vi "Final_LP2.vi"() -> ()   [LabVIEW 2017]
panel:
  out "Waveform Chart":cluster{"TEM1":dbl, "TEM2":dbl, "TEM2":dbl}(graph)
  out "IsOpen 3":bool
  out "Multicolumn Listbox":i32(listbox)
  out "LED 3":bool
  out "LED 2":bool
  out "LED 1":bool
  in  "PUERTO":string(combo)
  in  "BaudRate":i32=9600
  in  "Close":bool
  in  "Open":bool
  in  "Umbral min3":dbl
  in  "Umbral max3":dbl
  in  "Umbral min2":dbl
  in  "Umbral max2":dbl
  in  "Umbral min1":dbl
  in  "Umbral max1":dbl
  out "lm35_3":dbl(knob) scale=0.0..150.0
  out "lm35_2":dbl(knob) scale=0.0..150.0
  out "lm35":dbl(knob) scale=0.0..150.0
  out "Sensor3_Dec":dbl
  out "Sensor2_Dec":dbl
  out "Sensor1_Dec":dbl
  out "element":string
  out "Datos":string
  out "BytesToRead":i32
  in  "STOP":bool
  # "PRUEBAS"
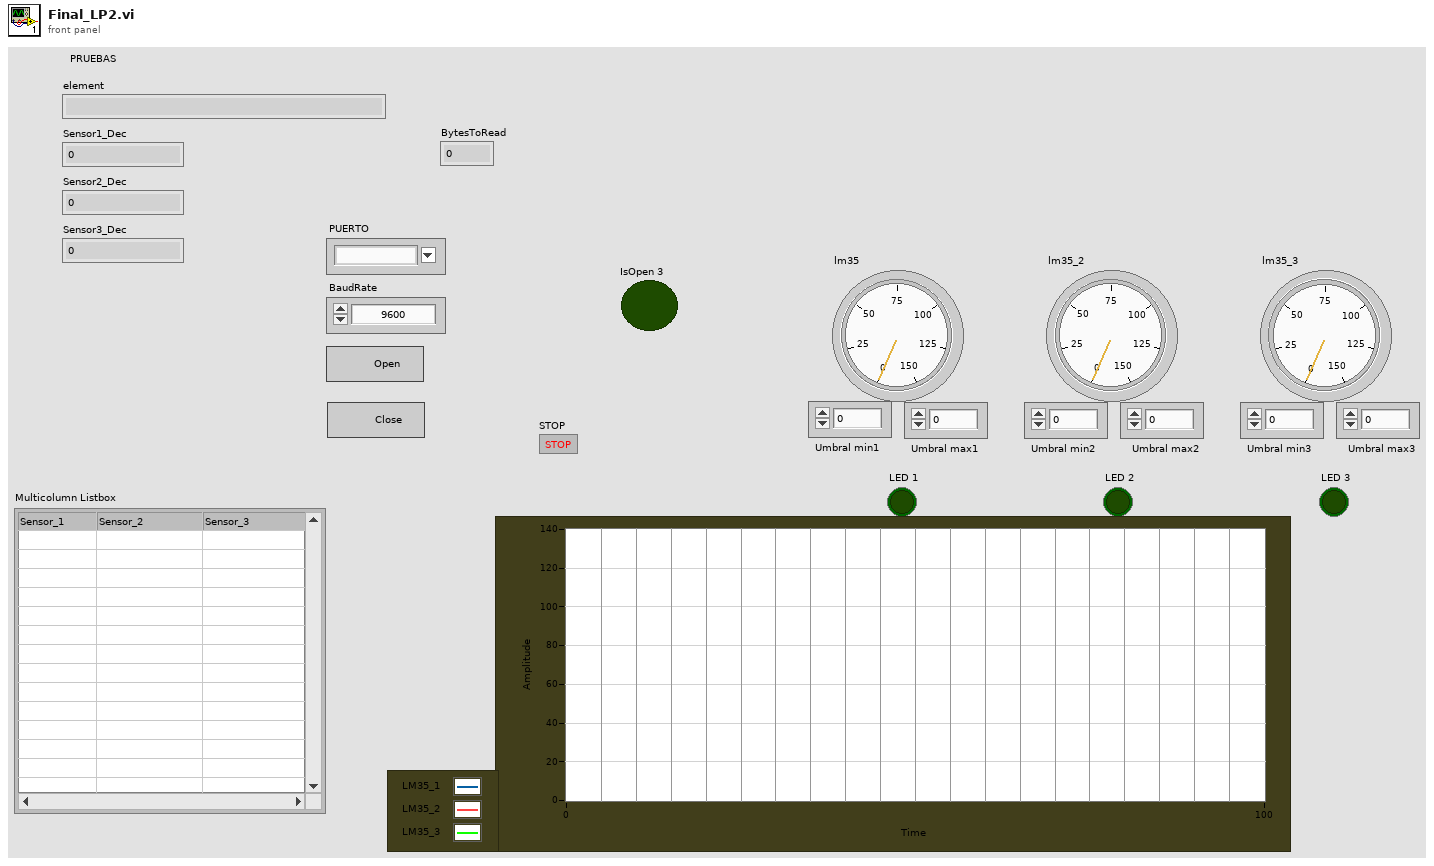
[diagram p1: front panel]
types:
  T1 = enum16{"open", "replace", "create", "open or create", "replace or create", "replace or create with confirmation"}
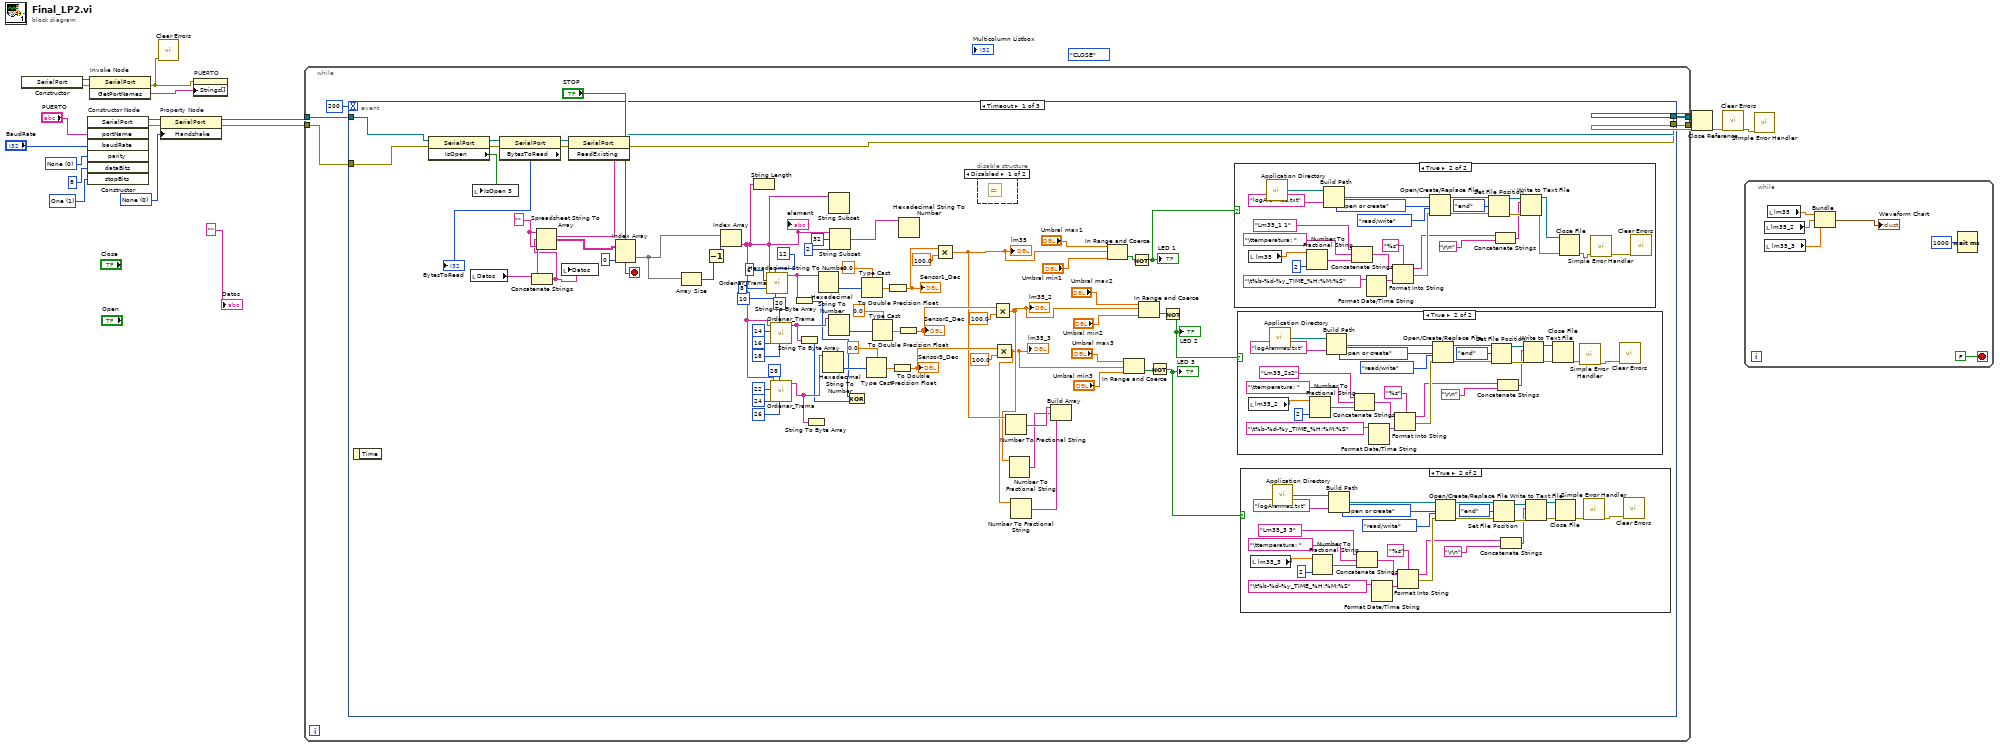
[diagram p0: block diagram]
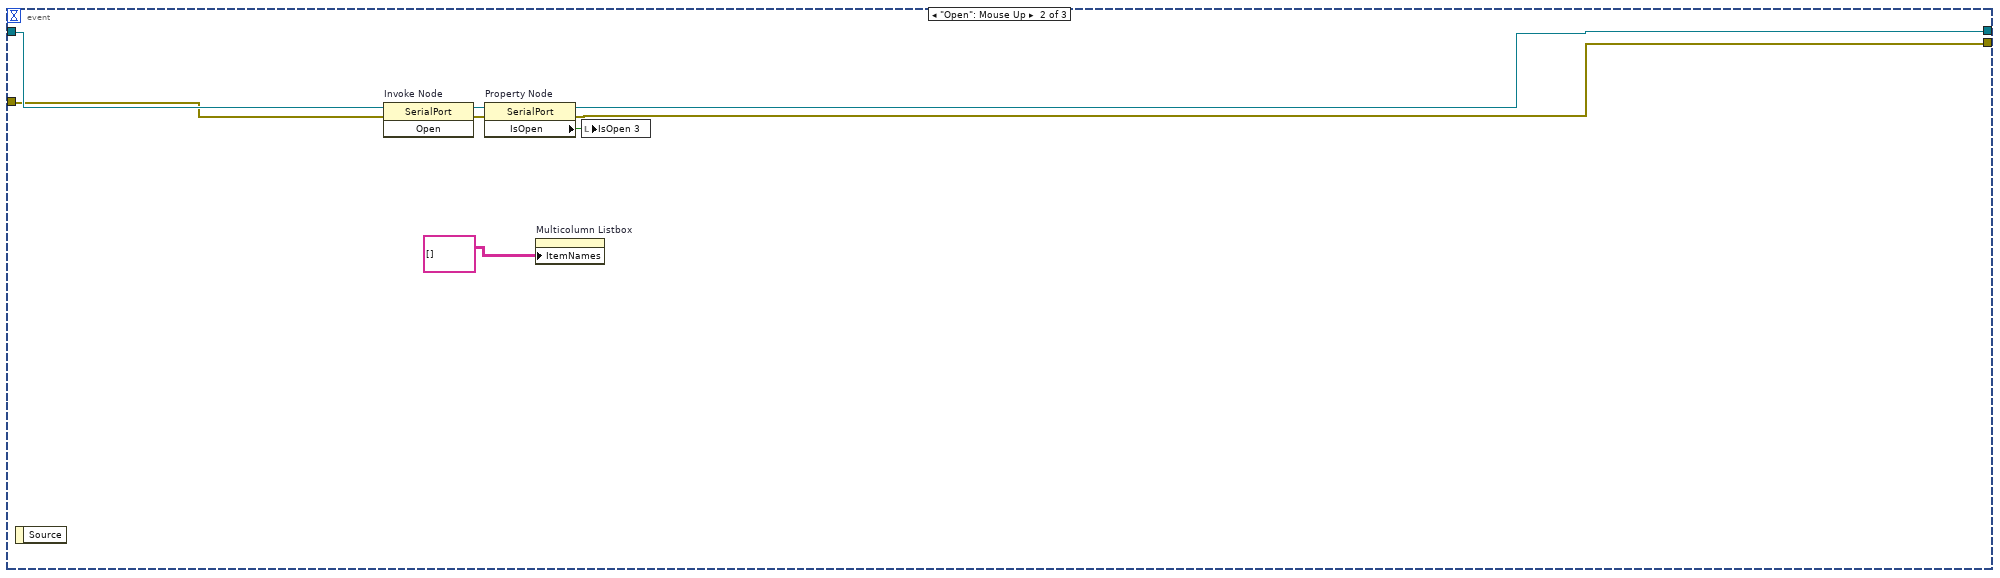
[diagram p6: hidden frame]
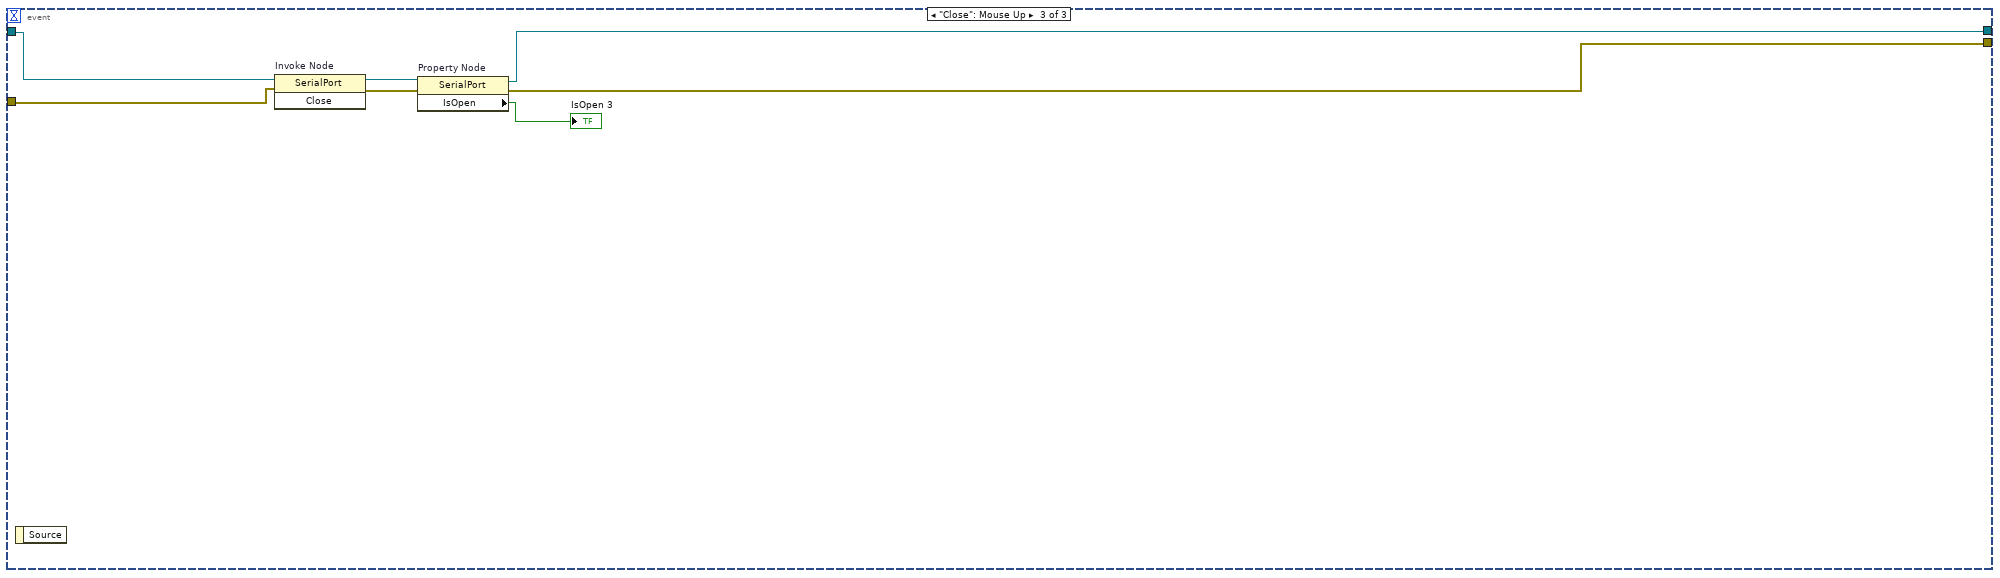
[diagram p7: hidden frame]
diagram:
  (unwired) enum16{"OPEN", "CLOSE", "READ"}."CLOSE"
  w10 = 1 items=["None", "One", "Two", "OnePointFive"] ("stopBits")
  w13 = 0 items=["None", "XOnXOff", "RequestToSend", "RequestToSendXOnXOff"] ("Handshake")
  w12 = 0 items=["None", "Odd", "Even", "Mark", "Space"] ("parity")
  n1 = constructor class="SerialPort"() -> (reference out=w17:refnum<k24>, error out=w16:errorcluster)  [unwired: 3 in, 1 out]
  n2 = constructor on="Constructor Node" class="SerialPort"("portName"="PUERTO", "baudRate"="BaudRate", "parity"=w12, "dataBits"=8, "stopBits"=w10) -> (reference out=w15:refnum<k24>, error out=w14:errorcluster)  [unwired: 3 in, 6 out]
  n3 = invoke on="Invoke Node" class="SerialPort" method="GetPortNames"(reference=w17, error in=w16) -> (error out=w7:errorcluster, "GetPortNames"=w8:string[])  [unwired: 1 in, 1 out]
  n4 = call <vilib>:"Clear Errors.vi"("error in (no error)"=w7) -> ()  [unwired: 5 in, 2 out]
  n5 = property on="Property Node" class="SerialPort"(reference=w15, error in=w14, "Handshake"=w13) -> (reference out=w5:refnum<k24>, error out=w4:errorcluster)
  n6 = property on="PUERTO" class="CmbBox"(error in=w7, "Strings[]"=w8) -> ()  [unwired: 1 in, 2 out]
  n7 = while {
    tunnel: w5 -> [w25]
    tunnel: [w21] -> w3
    tunnel: w4 -> [w24]
    tunnel: [w20] -> w2
    stop <- "STOP" stop-if-true
    n8 = event shown="[0] Timeout" {
      selector: _ -> [_ _ _]
      dyn-events: _ -> [_ _ _]
      timeout: 200 -> [_ _ _]
      tunnel: [w98 w182 w189] -> w21
      tunnel: w25 -> [w97 w184 w191]
      tunnel: w24 -> [w96 w183 w190]
      tunnel: [w95 w181 w188] -> w20
      event Timeout {
        w91 = "" ("format string")
        n9 = event-data() -> ()  [unwired: 1 in, 1 out]
        n10 = property class="SerialPort"(reference=w97, error in=w96) -> (reference out=w42:refnum<k24>, error out=w41:errorcluster, "IsOpen"=w40:bool)
        n11 = local read "Datos"() -> (w89:string)
        n12 = local write "IsOpen 3"(w40) -> ()
        n13 = property class="SerialPort"(reference=w42, error in=w41) -> (reference out=w92:refnum<k24>, error out=w94:errorcluster, "BytesToRead"=→"BytesToRead":i32)
        n14 = invoke class="SerialPort" method="ReadExisting"(reference=w92, error in=w94) -> (reference out=w98:refnum<k24>, error out=w95:errorcluster, "ReadExisting"=w90:string)  [unwired: 1 in]
        n15 = Concatenate Strings(w89, w90) -> (w88:string)
        n16 = Spreadsheet String To Array(format string=w91, spreadsheet string=w88, array type (2D Dbl)=w91) -> (array=w87:string[][])  [unwired: 1 in]
        n17 = local write "Datos"(w88) -> ()
        n18 = Index Array(array=w87, index (col)=0 ("disabled index (col)")) -> (element=w85:string[])  [unwired: 1 in]
        n19 = Array Size(array=w85) -> (size(s)=w84:i32)
        n20 = Decrement(x=w84) -> (x-1=w83:i32)
        n21 = Index Array(array=w85, index=w83) -> (element=w43:string)
        "element" <- w43
        n22 = String Length(string=w43) -> ()  [unwired: 1 out]
        n23 = call "Ordenar_Trama.vi"("offset (0) 3"=10 ("offset (0)"), "offset (0) 4"=12 ("offset (0)"), "offset (0) 2"=8 ("offset (0)"), "offset (0) 1"=6 ("offset (0)"), "format string"=w43) -> ("String"=w39:string)  [unwired: 6 in]
        n24 = call "Ordenar_Trama.vi"("offset (0) 3"=18, "offset (0) 4"=20, "offset (0) 2"=16, "offset (0) 1"=14, "format string"=w43) -> ("String"=w38:string)  [unwired: 6 in]
        n25 = call "Ordenar_Trama.vi"("offset (0) 3"=26, "offset (0) 4"=28, "offset (0) 2"=24, "offset (0) 1"=22, "format string"=w43) -> ("String"=w37:string)  [unwired: 6 in]
        n26 = String To Byte Array(string=w39) -> (unsigned byte array=w36:u8[])
        n27 = String To Byte Array(string=w38) -> (unsigned byte array=w35:u8[])
        n28 = String To Byte Array(string=w37) -> ()  [unwired: 1 out]
        n29 = Hexadecimal String To Number(string=w39) -> (number=w70:u32)  [unwired: 2 in, 1 out]
        n30 = Hexadecimal String To Number(string=w37) -> (number=w64:u32)  [unwired: 2 in, 1 out]
        n31 = String Subset(string=w43) -> ()  [unwired: 2 in, 1 out]
        n32 = Hexadecimal String To Number(string=w38) -> (number=w65:u32)  [unwired: 2 in, 1 out]
        n33 = String Subset(string=w43, offset (0)=32, length (rest)=2 ("length (rest)")) -> (substring=w44:string)
        n34 = Exclusive Or(1:w35, 2:w36) -> ()  [unwired: 1 out]
        n35 = Type Cast(type=sgl 0.0, x=w70) -> (*(type *) &x=w68:sgl)
        n36 = Type Cast(type=sgl 0.0, x=w64) -> (*(type *) &x=w62:sgl)
        n37 = Type Cast(type=sgl 0.0, x=w65) -> (*(type *) &x=w67:sgl)
        n38 = To Double Precision Float(number=w68) -> (double precision float=w61:dbl)
        "Sensor1_Dec" <- w61
        n39 = To Double Precision Float(number=w62) -> (double precision float=w57:dbl)
        "Sensor3_Dec" <- w57
        n40 = To Double Precision Float(number=w67) -> (double precision float=w56:dbl)
        "Sensor2_Dec" <- w56
        n41 = Hexadecimal String To Number(string=w44) -> ()  [unwired: 2 in, 2 out]
        n42 = Multiply(x=w61, y=100.0) -> (x*y=w31:dbl)
        "lm35" <- w31
        n43 = disable-structure shown="Disabled" {
          frame Disabled {
            n44 = Equal?() -> ()  [unwired: 2 in, 1 out]
          }
          frame Enabled {
          }
        }
        n45 = Multiply(x=w56, y=100.0) -> (x*y=w30:dbl)
        "lm35_2" <- w30
        n46 = Multiply(x=w57, y=100.0) -> (x*y=w29:dbl)
        "lm35_3" <- w29
        n47 = Number To Fractional String(number=w31) -> (F-format string=w28:string)  [unwired: 3 in]
        n48 = Number To Fractional String(number=w30) -> (F-format string=w27:string)  [unwired: 3 in]
        n49 = Number To Fractional String(number=w29) -> (F-format string=w26:string)  [unwired: 3 in]
        n50 = Build Array(w28, w27, w26) -> ()  [unwired: 1 out]
        n51 = In Range and Coerce(upper limit="Umbral max1", x=w31, lower limit="Umbral min1") -> (In Range?=w49:bool)  [unwired: 1 out]
        n52 = In Range and Coerce(upper limit="Umbral max3", x=w29, lower limit="Umbral min3") -> (In Range?=w47:bool)  [unwired: 1 out]
        n53 = Not(x=w49) -> (.not. x?=w34:bool)
        "LED 1" <- w34
        n54 = In Range and Coerce(upper limit="Umbral max2", x=w30, lower limit="Umbral min2") -> (In Range?=w48:bool)  [unwired: 1 out]
        n55 = Not(x=w47) -> (.not. x?=w32:bool)
        "LED 3" <- w32
        n56 = Not(x=w48) -> (.not. x?=w33:bool)
        "LED 2" <- w33
        n57 = case shown="True" w34 {
          frame False {
          }
          frame True {
            n58 = local read "lm35"() -> (w157:dbl)
            n59 = call <vilib>:"Application Directory.vi"() -> ("Application Directory"=w179:path)
            n60 = Number To Fractional String(number=w157, precision (6)=i16 2) -> (F-format string=w160:string)  [unwired: 2 in]
            n61 = Build Path(base path=w179, name or relative path="logAlarmas.txt") -> (appended path=w178:path)
            n62 = Concatenate Strings("Lm35_1 1" ("format string"), "\ttemperatura: " ("format string"), w160) -> (w159:string)
            n63 = Format Date/Time String(time format string (%c)="\t%b-%d-%y_TIME_%H:%M:%S") -> (date/time string=w166:string)  [unwired: 2 in]
            n64 = Format Into String(format string="%s", initial string=w159, w166) -> (resulting string=w164:string, error out=w168:errorcluster)  [unwired: 1 in]
            n65 = Open/Create/Replace File(file path (use dialog)=w178, error in=w168, operation (0:open)=T1."open or create", access (0:read/write)=enum16{"read/write", "read-only", "write-only"}."read/write") -> (refnum out=w174:refnum<file>, error out=w173:errorcluster)  [unwired: 2 in, 1 out]
            n66 = Set File Position(refnum=w174, from (0:start)=enum16{"start", "end", "current"}."end", error in=w173) -> (refnum out=w171:refnum<file>, error out=w170:errorcluster)  [unwired: 1 in]
            n67 = Concatenate Strings(w164, "\r\n") -> (w163:string)
            n68 = Write to Text File(file (use dialog)=w171, text=w163, error in=w170) -> (refnum out=w156:refnum<file>, error out=w155:errorcluster)  [unwired: 1 in, 1 out]
            n69 = Close File(refnum=w156, error in=w155) -> (error out=w154:errorcluster)  [unwired: 1 out]
            n70 = call <vilib>:"Simple Error Handler.vi"("error in (no error)"=w154) -> ("error out"=w153:errorcluster)  [unwired: 4 in, 4 out]
            n71 = call <vilib>:"Clear Errors.vi"("error in (no error)"=w153) -> ()  [unwired: 5 in, 2 out]
          }
        }
        n72 = case shown="True" w33 {
          frame False {
          }
          frame True {
            n73 = local read "lm35_2"() -> (w128:dbl)
            n74 = call <vilib>:"Application Directory.vi"() -> ("Application Directory"=w152:path)
            n75 = Number To Fractional String(number=w128, precision (6)=i16 2) -> (F-format string=w131:string)  [unwired: 2 in]
            n76 = Build Path(base path=w152, name or relative path="logAlarmas.txt") -> (appended path=w151:path)
            n77 = Concatenate Strings("Lm35_2s2" ("format string"), "\ttemperatura: " ("format string"), w131) -> (w130:string)
            n78 = Format Date/Time String(time format string (%c)="\t%b-%d-%y_TIME_%H:%M:%S") -> (date/time string=w137:string)  [unwired: 2 in]
            n79 = Format Into String(format string="%s", initial string=w130, w137) -> (resulting string=w135:string, error out=w139:errorcluster)  [unwired: 1 in]
            n80 = Open/Create/Replace File(file path (use dialog)=w151, error in=w139, operation (0:open)=T1."open or create", access (0:read/write)=enum16{"read/write", "read-only", "write-only"}."read/write") -> (refnum out=w147:refnum<file>, error out=w146:errorcluster)  [unwired: 2 in, 1 out]
            n81 = Set File Position(refnum=w147, from (0:start)=enum16{"start", "end", "current"}."end", error in=w146) -> (refnum out=w144:refnum<file>, error out=w143:errorcluster)  [unwired: 1 in]
            n82 = Concatenate Strings(w135, "\r\n") -> (w134:string)
            n83 = Write to Text File(file (use dialog)=w144, text=w134, error in=w143) -> (refnum out=w142:refnum<file>, error out=w141:errorcluster)  [unwired: 1 in, 1 out]
            n84 = Close File(refnum=w142, error in=w141) -> (error out=w126:errorcluster)  [unwired: 1 out]
            n85 = call <vilib>:"Simple Error Handler.vi"("error in (no error)"=w126) -> ("error out"=w127:errorcluster)  [unwired: 4 in, 4 out]
            n86 = call <vilib>:"Clear Errors.vi"("error in (no error)"=w127) -> ()  [unwired: 5 in, 2 out]
          }
        }
        n87 = case shown="True" w32 {
          frame False {
          }
          frame True {
            n88 = local read "lm35_3"() -> (w101:dbl)
            n89 = call <vilib>:"Application Directory.vi"() -> ("Application Directory"=w125:path)
            n90 = Number To Fractional String(number=w101, precision (6)=i16 2) -> (F-format string=w104:string)  [unwired: 2 in]
            n91 = Build Path(base path=w125, name or relative path="logAlarmas.txt") -> (appended path=w124:path)
            n92 = Concatenate Strings("Lm35_3 3" ("format string"), "\ttemperatura: " ("format string"), w104) -> (w103:string)
            n93 = Format Date/Time String(time format string (%c)="\t%b-%d-%y_TIME_%H:%M:%S") -> (date/time string=w110:string)  [unwired: 2 in]
            n94 = Format Into String(format string="%s", initial string=w103, w110) -> (resulting string=w108:string, error out=w112:errorcluster)  [unwired: 1 in]
            n95 = Open/Create/Replace File(file path (use dialog)=w124, error in=w112, operation (0:open)=T1."open or create", access (0:read/write)=enum16{"read/write", "read-only", "write-only"}."read/write") -> (refnum out=w120:refnum<file>, error out=w119:errorcluster)  [unwired: 2 in, 1 out]
            n96 = Set File Position(refnum=w120, from (0:start)=enum16{"start", "end", "current"}."end", error in=w119) -> (refnum out=w117:refnum<file>, error out=w116:errorcluster)  [unwired: 1 in]
            n97 = Concatenate Strings(w108, "\r\n") -> (w107:string)
            n98 = Write to Text File(file (use dialog)=w117, text=w107, error in=w116) -> (refnum out=w115:refnum<file>, error out=w114:errorcluster)  [unwired: 1 in, 1 out]
            n99 = Close File(refnum=w115, error in=w114) -> (error out=w99:errorcluster)  [unwired: 1 out]
            n100 = call <vilib>:"Simple Error Handler.vi"("error in (no error)"=w99) -> ("error out"=w100:errorcluster)  [unwired: 4 in, 4 out]
            n101 = call <vilib>:"Clear Errors.vi"("error in (no error)"=w100) -> ()  [unwired: 5 in, 2 out]
          }
        }
      }
      event "Open": Mouse Up {
        n102 = event-data() -> ()  [unwired: 1 in, 1 out]
        n103 = invoke on="Invoke Node" class="SerialPort" method="Open"(reference=w184, error in=w183) -> (reference out=w186:refnum<k24>, error out=w185:errorcluster)  [unwired: 1 in, 1 out]
        n104 = property on="Property Node" class="SerialPort"(reference=w186, error in=w185) -> (reference out=w182:refnum<k24>, error out=w181:errorcluster, "IsOpen"=w180:bool)
        n105 = property on="Multicolumn Listbox" class="MCListbox (strict)"("ItemNames"=string[][] []) -> ()  [unwired: 2 in, 2 out]
        n106 = local write "IsOpen 3"(w180) -> ()
      }
      event "Close": Mouse Up {
        n107 = event-data() -> ()  [unwired: 1 in, 1 out]
        n108 = invoke on="Invoke Node" class="SerialPort" method="Close"(reference=w191, error in=w190) -> (reference out=w194:refnum<k24>, error out=w193:errorcluster)  [unwired: 1 in, 1 out]
        n109 = property on="Property Node" class="SerialPort"(reference=w194, error in=w193) -> (reference out=w189:refnum<k24>, error out=w188:errorcluster, "IsOpen"=→"IsOpen 3":bool)
      }
    }
  }
  n110 = Close Reference(reference=w3, error in (no error)=w2) -> (error out=w19:errorcluster)
  n111 = call <vilib>:"Clear Errors.vi"("error in (no error)"=w19) -> ("error out"=w18:errorcluster)  [unwired: 5 in, 1 out]
  n112 = while {
    stop <- FALSE stop-if-true
    n113 = local read "lm35_2"() -> (w198:dbl)
    n114 = local read "lm35_3"() -> (w197:dbl)
    n115 = local read "lm35"() -> (w199:dbl)
    n116 = Bundle("lm35"=w199, "lm35_2"=w198, "lm35_3"=w197) -> (→"Waveform Chart":cluster{"lm35":dbl, "lm35_2":dbl, "lm35_3":dbl})  [unwired: 1 in]
    n117 = Wait (ms)(milliseconds to wait=u32 1000) -> ()  [unwired: 1 out]
  }
  n118 = call <vilib>:"Simple Error Handler.vi"("error in (no error)"=w18) -> ()  [unwired: 1 in, 8 out]
  "Datos" <- "" ("Datos")
